vi "Get All Combinations of Array.vi"(8 "error in (no error)":errorcluster, 9 "Combination Length":i32, 11 "Array":i32[](array[numeric])) -> (0 "error out":errorcluster, 2 "Enough Points":bool, 3 "Results Out":i32[][](array[numeric]))   [LabVIEW 2011]
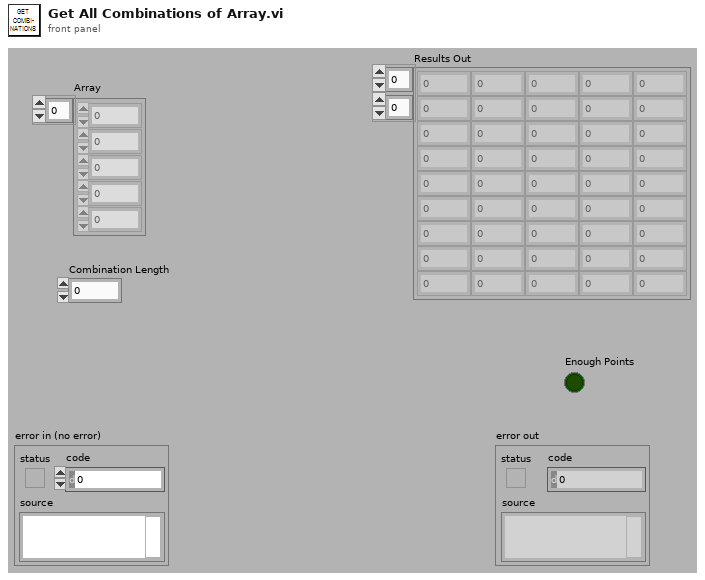
[diagram p1: front panel]
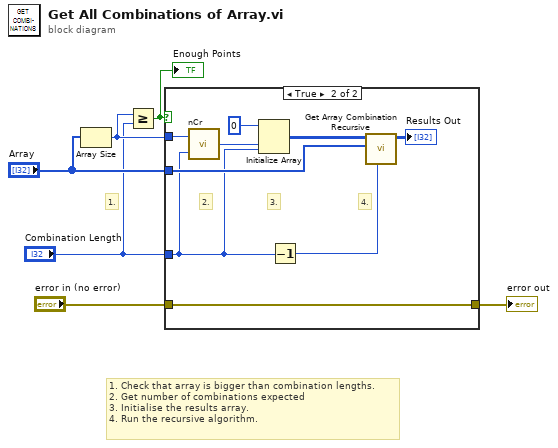
[diagram p0: block diagram]
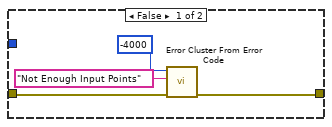
[diagram p2: hidden frame]
diagram:
  # "1. Check that array is bigger than combination lengths.\n2. Get number of combinations expected\n3. Initialise the results array.\n4. Run the recursive algorithm."
  # "1."
  n1 = Array Size(array="Array") -> (size(s)=w5:i32)
  n2 = Greater Or Equal?(x=w5, y="Combination Length") -> (x >= y?=w3:bool)
  "Enough Points" <- w3
  n3 = case shown="True" w3 {
    tunnel: "Array" -> [_ w16]
    tunnel: w5 -> [_ w13]
    tunnel: "Combination Length" -> [_ w12]
    tunnel: [w9 w11] -> w2
    tunnel: "error in (no error)" -> [w10 w11]
    frame False {
      n4 = call <vilib>:"Error Cluster From Error Code.vi"("error in (no error)"=w10, "error message (\"\")"="Not Enough Input Points" ("error message (\"\")"), "error code (0)"=-4000) -> ("error out"=w9:errorcluster)  [unwired: 6 in]
    }
    frame True {
      # "4."
      # "3."
      # "2."
      n5 = call "nCr.vi"("R"=w12, "N"=w13) -> ("Combinations"=w18:i32)
      n6 = Initialize Array(0 ("Combination Length"), w18, w12) -> (w17:i32[][])
      n7 = Decrement(x=w12) -> (x-1=w15:i32)
      n8 = call "Get Array Combination Recursive.vi"("Max Column Index"=w15, "Array"=w16, "Results"=w17) -> ("Results Out"=→"Results Out":i32[][])  [unwired: 7 in, 1 out]
    }
  }
  "error out" <- w2
